vi "Dispose Lock.vi"(8 "error in (no error)":errorcluster, 11 "Protected Pointer in":refnum<class "Protected Pointer.lvclass">) -> (0 "error out":errorcluster, 3 "Protected Pointer out":refnum<class "Protected Pointer.lvclass">)   [LabVIEW 2017, in "Protected Pointer.lvclass"]
uses:
  Protected Pointer.lvclass
  Invalid Lock.vi
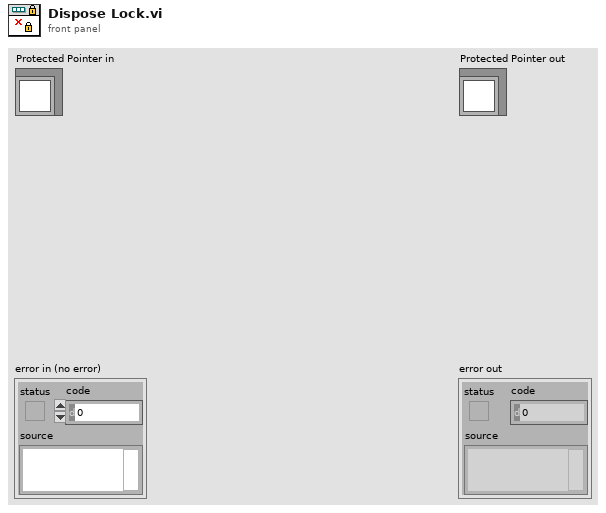
[diagram p1: front panel]
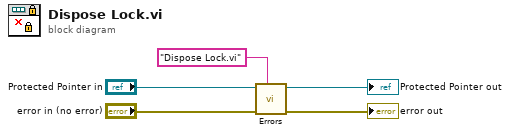
[diagram p0: block diagram]
diagram:
  n1 = call-poly "Errors.vi"("source vi name"="Dispose Lock.vi", "error in (no error)"="error in (no error)", "Lockable Pointer in"="Protected Pointer in") -> ("error out"=→"error out":errorcluster, "Lockable Pointer out"=→"Protected Pointer out":refnum<class "Protected Pointer.lvclass">)  [unwired: 7 in]
